vi "Empty Array.vi"(2 "Cluster":cluster{"Vfast":dbl[], "Decimated Array":dbl[]}) -> (7 "Boolean":bool)   [LabVIEW 2016]
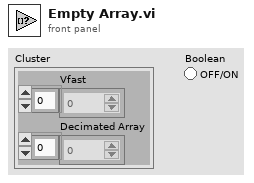
[diagram p1: front panel]
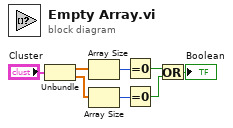
[diagram p0: block diagram]
diagram:
  n1 = Unbundle("Cluster") -> ("Vfast"=w2:dbl[], "Decimated Array"=w3:dbl[])
  n2 = Array Size(array=w2) -> (size(s)=w4:i32)
  n3 = Array Size(array=w3) -> (size(s)=w5:i32)
  n4 = Equal To 0?(x=w4) -> (x = 0?=w6:bool)
  n5 = Equal To 0?(x=w5) -> (x = 0?=w7:bool)
  n6 = Or(x=w6, y=w7) -> (x .or. y?=→"Boolean":bool)
